vi "ArrangeNodes Main.vi"(1 "localVariablesOut":T1 {"ObjectHotspots"."HotSpot"."y" format="%.2f"; "ObjectHotspots"."HotSpot"."x" format="%.2f"; "NodesBounds"."height" format="%.2f"; "NodesBounds"."width" format="%.2f"; "NodesBounds"."y" format="%.2f"; "NodesBounds"."x" format="%.2f"; "offset"."y" format="%.2f"; "offset"."x" format="%.2f"; "gridSize" format="%.2f"; "dragStartBounds"."height" format="%.2f"; "dragStartBounds"."width" format="%.2f"; "dragStartBounds"."y" format="%.2f"; "dragStartBounds"."x" format="%.2f"; "dragStartPoint"."y" format="%.2f"; "dragStartPoint"."x" format="%.2f"; "rubberBandStart"."y" format="%.2f"; "rubberBandStart"."x" format="%.2f"; "lastMousePoint"."y" format="%.2f"; "lastMousePoint"."x" format="%.2f"; "zoom" format="%.2f"}) -> (15 "Cancel":bool)   [LabVIEW 2014]
uses:
  <resource>/Framework/Providers/Open_GDS/UML/UMLEditor/UMLEditor LocalVariablesType.ctl
  <resource>/Framework/Providers/Open_GDS/UML/Graphics_class/Graphics.lvclass
  <resource>/Framework/Providers/Open_GDS/UML/Grid_class/Grid.lvclass
  <resource>/Framework/Providers/Open_GDS/UML/AbstractEdge_class/AbstractEdge.lvclass
  <resource>/Framework/Providers/Open_GDS/UML/AbstractNode_class/AbstractNode.lvclass
  <resource>/Framework/Providers/Open_GDS/UML/UMLEditor/UMLEditor statesType.ctl
  <resource>/Framework/Providers/Open_GDS/UML/UMLEditor/UMLEditor tooltype.ctl
  <resource>/Framework/Providers/Open_GDS/UML/UMLEditor/UMLEditor toolsType.ctl
  <resource>/Framework/Providers/Open_GDS/UML/UMLEditor/UMLEditor_DiagramInfo.ctl
  <resource>/Framework/Providers/Open_GDS/UML/Graph_class/Graph.lvclass
  <resource>/Framework/Providers/Open_GDS/UML/General/Point/Point Point2D.ctl
  <resource>/Framework/Providers/Open_GDS/UML/General/Rectangle/Rectangle Rectangle2D.ctl
  <resource>/Framework/Providers/Open_GDS/UML/UMLEditor/UMLEditor ExportType.ctl
  <resource>/Framework/Providers/Open_GDS/UML/UMLEditor/UMLEditor FlattenCommandType.ctl
  <resource>/Framework/Providers/Open_GDS/UML/UMLEditor/UMLEditor ExecuteCommandType.ctl
  <resource>/Framework/Providers/Open_GDS/UML/ContextHelp/ContextHelp_EventType.ctl
  <resource>/Framework/Providers/Open_GDS/UML/UMLEditor/UMLEditor_HotSpotData.ctl
  <resource>/Framework/Providers/Open_GDS/UML/UMLEditor/UMLEditor_HotSpotType.ctl
  <resource>/Framework/Providers/Open_GDS/UML/UmlEditor_class/EventData.ctl
  <resource>/Framework/Providers/Open_GDS/UML/ArrangeNodes/private/ArrangeNodes LocalVar.ctl
  <resource>/Framework/Providers/Open_GDS/UML/ClassNode_class/ClassNode.lvclass
  <resource>/Framework/Providers/Open_GDS/UML/InterfaceNode_class/InterfaceNode.lvclass
  <resource>/Framework/Providers/Open_GDS/UML/StateNode_class/StateNode.lvclass
  <resource>/Framework/Providers/Open_GDS/UML/ContextHelp/ContextHelp_HelpTexts.ctl
  <resource>/Framework/Providers/Open_GDS/UML/MultiLineString_class/MultiLineString.lvclass
  <resource>/Framework/Providers/Open_GDS/UML/UmlEditor_class/UmlEditor.lvclass
panel:
  out "Picture":picture
  in  "Shake":bool
  in  "Help":bool
  in  "Zoom":enum16{"Normal", "Small", "Smaller", "Smallest"}(ring)
  in  "Auto Zoom":bool=TRUE
  in  "decrease":bool
  in  "OK":bool
  in  "Max Length":i32=350 min=10 max=1000
  in  "Min Length":i32=50 min=10 max=1000
  in  "increase":bool
  in  "shorten":bool
  in  "cancel":bool
  # "Left-Click and drag\na class.\n\nRight-click to lock/\nunlock class."
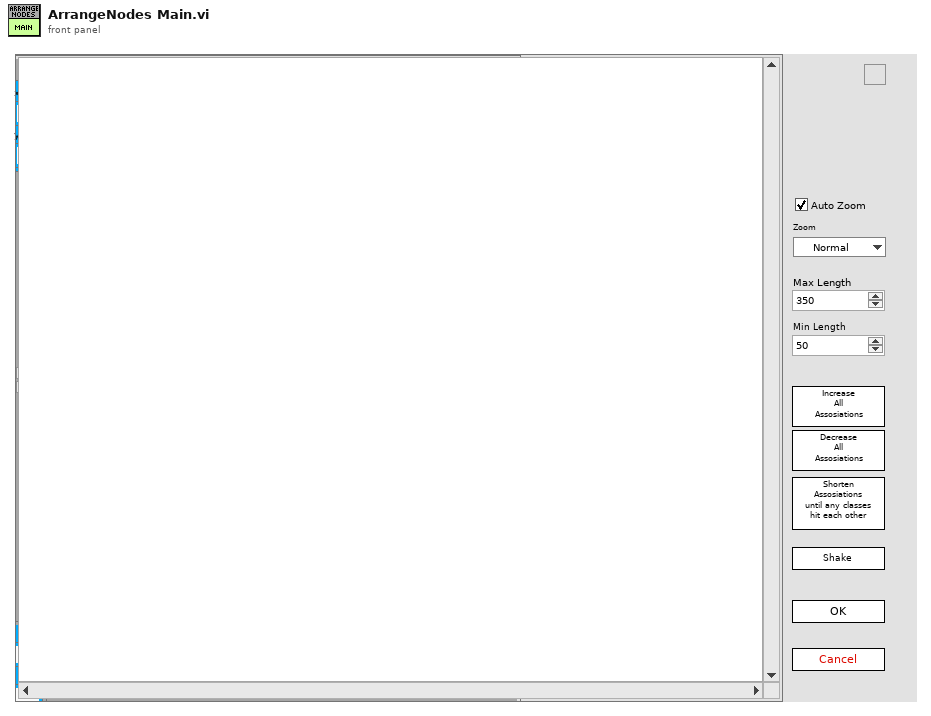
[diagram p1: front panel]
types:
  T1 = typedef "UMLEditor LocalVariablesType.ctl" = cluster{"state":T2, "graphics":refnum<class "Graphics.lvclass">, "grid":refnum<class "Grid.lvclass">, "toolType":T3, "tool":T4, "diagramIndex":i32, "diagrams":T5[], "zoom":dbl, "hideGrid":bool, "lastMousePoint":T6, "rubberBandStart":T6, "dragStartPoint":T6, "dragStartBounds":T7, "gridColor":u32, "gridSize":dbl, "CONNECT_THRESHOLD":i32, "selcted":T3, "selectedEdge":refnum<class "AbstractEdge.lvclass">, "butDwn":bool, "lastPress":u32, "modified":bool, "offset":T6, "menu":refnum<k9>, "file":path, "saveAs":bool, "newSelected":bool, "exportype":T8, "quit":bool, "revHistory":cluster{"rev":string, "text":string}[], "FlattenCommandSettings":T9, "PopUpMessageEvent":T11, "ResizePanelInProgress":bool, "NodesBounds":T7, "ToolHelp":bool, "ViRef":refnum<vi>, "FP_CtrlEnterEvents":refnum<event-registration>, "SelectedNodes":refnum<class "AbstractNode.lvclass">[], "mouse":refnum<k1>, "RevPlugInPath":path, "Action":string, "KeyPressTime":u32, "Cursors":refnum<k1>[], "ObjectHotspots":T12[], "HotSpotCursor":bool, "HotSpotFunction":T13, "Don'tDeleteChildren":bool, "ShiftDown":bool, "CtrlDown":bool, "HotSpotNode":refnum<class "AbstractNode.lvclass">, "Sync":bool, "SyncTime":u32, "ForceSyncNow":bool, "LastSync":timestamp, "XMI_Import":bool, "Event":refnum<event-registration>}
  T2 = typedef "UMLEditor statesType.ctl" = enum16{"Idle", "CheckLicense", "revHistory", "Init", "Init2", "EditSelected", "RemoveSelected", "PaintComponent", "ChangeZoom", "ChangeGridSize", "Open", "Close", "Save", "ExportPicture", "Export", "Repaint", "Error", "Exit", "QUIT", "CreateScript", "ExecuteScript", "ClassReversedEngineering", "PlugInReverseEngineering", "StateReversedEngineering", "AutoPlace", "ExecuteCommand", "OpenClass", "SyncAll", "StraightenAssociation", "Copy", "Paste", "AddNodeFromProjectTree", "AddNodeFromProjectTree+SyncAll", "PanAndRepaint", "Init3", "CopyPaste", "ApplyDesignPattern", "AnalyseViInStateDiagram", "AutoSync"}
  T3 = typedef "UMLEditor tooltype.ctl" = enum16{"None", "Node", "Edge"}
  T4 = typedef "UMLEditor toolsType.ctl" = enum16{"CD_Select", "CD_Class", "CD_Interface", "CD_Package", "CD_Note", "CD_Dependency", "CD_Inheritance", "CD_InterfaceImp", "CD_Association", "CD_Aggregation", "CD_Composite", "CD_NoteConn", "SQD_Select", "SQD_Object", "SQD_ActionBar", "SQD_Note", "SQD_Call", "SQD_NoteConn", "UD_Select", "UD_System", "UD_Actor", "UD_UseCase", "UD_Note", "UD_Assoiciation", "UD_Generalization", "UD_GeneralizationIncludes", "UD_GeneralizationExtends", "UD_Realization", "UD_Relationship", "UD_NoteEdge", "STD_Select", "STD_State", "STD_InitailState", "STD_FinalState", "STD_ChoiseState", "STD_StateTransation", "STD_Note", "STD_NoteEdge", "DM_Select", "DM_VI", "DM_Module", "DM_Request", "DM_RequestWait", "DM_Roundtrip", "DM_Broadcast", "DM_Note", "DM_NoteEdge"}
  T5 = typedef "UMLEditor_DiagramInfo.ctl" = cluster{"name":string, "diagramType":string, "unsaved":bool, "graph":refnum<class "Graph.lvclass">, "saveDir":path}
  T6 = typedef "Point Point2D.ctl" = cluster{"x":dbl, "y":dbl}
  T7 = typedef "Rectangle Rectangle2D.ctl" = cluster{"x":dbl, "y":dbl, "width":dbl, "height":dbl}
  T8 = typedef "UMLEditor ExportType.ctl" = enum16{"None", "Printer", "png", "jpg", "roseUML"}
  T9 = typedef "UMLEditor FlattenCommandType.ctl" = cluster{"Command":T10, "CommandData":variant}
  T10 = typedef "UMLEditor ExecuteCommandType.ctl" = enum16{"SyncUmlFromCode", "SyncCodeFromUML", "OpenClass", "OpenFile", "CreateClass", "CreateVI", "OpenClassAttribute", "LocateInProject"}
  T11 = typedef "ContextHelp_EventType.ctl" = refnum<user-event>
  T12 = typedef "UMLEditor_HotSpotData.ctl" = cluster{"Node":refnum<class "AbstractNode.lvclass">, "HotSpot":T6, "Function":T13}
  T13 = typedef "UMLEditor_HotSpotType.ctl" = enum16{"N", "NE", "E", "SE", "S", "SW", "W", "NW", "Expand", "Collaps"}
  T14 = typedef "ArrangeNodes LocalVar.ctl" = cluster{"nodes":cluster{"x":dbl, "y":dbl, "w":dbl, "h":dbl, "dx":dbl, "dy":dbl, "fixed":bool, "text":string, "maxCornerDist":dbl}[], "edges":cluster{"from":i32, "to":i32, "len":dbl}[], "nodeSelected":i32, "drag":bool, "NodeRef":u32[], "DragStart":cluster{"X":i32, "Y":i32}, "fixedBeforeDrag":bool, "Cancel":bool, "ClassNodes":refnum<class "AbstractNode.lvclass">[]}
  T15 = cluster{"bounds":T7, "className":string, "nodeRef":refnum<class "AbstractNode.lvclass">}[]
  T16 = cluster{"index of element":i32, "index of element":i32, bool}[]
  T17 = typedef "ContextHelp_HelpTexts.ctl" = enum16{"None(Hide)", "Default", "Help", "Welcome", "GettingStarted", "ClassDiagram_Help", "SequenceDiagram_Help", "UseCaseDiagram_Help", "BSelect", "BClass", "BInterface", "BPackage", "BNote", "BDependency", "BInheritance", "BInterfaceImplementation", "BAssociation", "BAggregation", "BCompAggregation", "BNoteConnector", "BObject", "BActionBar", "BCall", "BSystem", "BActor", "BUseCase", "BGeneralization", "BIncludes", "BExtends", "BUseCaseDiagramAssociation", "ClassRelationshipEdge editDialog_Bent Style", "ClassRelationshipEdge editDialog_RelationType", "ClassRelationshipEdge editDialog_Reverse association", "ClassRelationshipEdge editDialog_Start label", "ClassRelationshipEdge editDialog_Middle label", "ClassRelationshipEdge editDialog_End label", "UMLEditor reversedEngineering_Pathes", "ReversedEngineering StateReverseDialog_Help", "ReversedEngineering StateQueuedSettings_Help", "UMLEditor reversedEngineering_AddTopVIs", "UMLEditor reversedEngineering_AddClasses", "UMLEditor reversedEngineering_AddDirs", "UMLEditor reversedEngineering_Recursively", "UMLEditor reversedEngineering_Remove", "UMLEditor reversedEngineering_ClearList", "UMLEditor reversedEngineering_HideSubAss", "UMLEditor reversedEngineering_CreateTypes", "UMLEditor reversedEngineering_OnlyInheritance", "UMLEditor reversedEngineering_CreateApplication", "UMLEditor reversedEngineering_OK", "UMLEditor reversedEngineering_Cancel", "UMLEditor reversedEngineering_Help", "UMLEditor createWizardScriptFile_ScriptfilePath", "UMLEditor createWizardScriptFile_ClassPath", "UMLEditor createWizardScriptFile_Use", "UMLEditor createWizardScriptFile_PrivateDirName", "UMLEditor createWizardScriptFile_DirAppend", "UMLEditor createWizardScriptFile_Separator Character", "UMLEditor createWizardScriptFile_OK", "UMLEditor createWizardScriptFile_Cancel", "UMLEditor createWizardScriptFile_Help", "ClassNode editDialog_Class Name", "InterfaceNode editDialog_Class Name", "ClassNode editDialog_Attribute", "ClassNode editDialog_Methods", "InterfaceNode editDialog_Methods", "ClassNode editDialog_connection", "InterfaceNode editDialog_connection", "ClassNode editDialog_StereoType", "ClassNode editDialog_ShowAttrib", "ClassNode editDialog_ShowMethods", "ClassNode editDialog_ClassPath", "ClassNode editDialog_AddAttribute", "ClassNode editDialog_AddMethod", "InterfaceNode editDialog_AddMethod", "ClassNode AttributeGuide_AttributeName", "ClassNode AttributeGuide_Array?", "ClassNode AttributeGuide_Data Type", "ClassNode AttributeGuide_RefName", "ClassNode AttributeGuide_Preview", "ClassNode AttributeGuide_OK", "ClassNode AttributeGuide_Cancel", "ClassNode MethodGuide_Visibility", "ClassNode MethodGuide_Method Name", "ClassNode MethodGuide_Preview", "ClassNode MethodGuide_OK", "ClassNode MethodGuide_Cancel", "CallNode EditCallProperties_AllButtons", "ObjectNode EditObjectlProperties_AllButtons", "ActorNode EditActorProperties_AllButtons", "UseCaseRelationshipNode EditUseCaselProperties_AllButtons", "UseCaseNode EditUseCaselProperties_AllButtons", "SystemNode EditSystemProperties_AllButtons", "ReversedEngineering UpdateAttributes_AllButtons", "StateNode editDialog_AllButtons", "StateTransition editDialog_AllButtons", "ArrangeNodes Main_Picture", "ArrangeNodes Main_Zoom", "ArrangeNodes Main_Auto Zoom", "ArrangeNodes Main_shorten", "ArrangeNodes Main_Min Length", "ArrangeNodes Main_Max Length", "ArrangeNodes Main_increase", "ArrangeNodes Main_decrease", "ArrangeNodes Main_Shake", "ArrangeNodes Main", "BState", "BInitialState", "BFinalState", "BStateTransition", "StateDiagram_Help", "StateDiagram_PropertiesAllButtons", "ReversedEngineering StateReverseDialog_ClearStates", "ReversedEngineering StateReverseDialog_UseQueuedStateMachines", "ReversedEngineering StateReverseDialog_QueuedSettings", "ReversedEngineering StateReverseDialog_SearchForVIs", "ReversedEngineering StateReverseDialog_SearchCriteria", "OptionsDialog_ClassBasePath", "OptionsDialog_VIPath", "OptionsDialog_ApplicationPath", "OptionsDialog_WizDir", "OptionsDialog_IniFilePath", "OptionsDialog_DefineColors", "OptionsDialog_Help", "OptionsDialog_CreateTypes", "ClassRelationshipEdge editDialog_SplitWire"}
  T18 = cluster{"bounds":T7, "text":string, "reference out":refnum<class "AbstractNode.lvclass">}
  T19 = cluster{"bounds":T7, "text":string, "reference out":refnum<class "AbstractNode.lvclass">}[]
  T20 = cluster{"x":dbl, "y":dbl, "w":dbl, "h":dbl, "dx":dbl, "dy":dbl, "fixed":bool, "text":string, "maxCornerDist":dbl}[]
  T21 = cluster{"x":dbl, "y":dbl, "w":dbl, "h":dbl, "dx":dbl, "dy":dbl, "fixed":bool, "text":string, "maxCornerDist":dbl}
  T22 = cluster{"index of element":i32, "index of element":i32, "isInheritance":bool}
  T23 = cluster{"index of element":i32, "index of element":i32, "isInheritance":bool}[]
  T24 = typedef "LVMouseTypeDef.ctl" = cluster{"Mouse Position":cluster{"X":i32, "Y":i32}, "Mouse Modifiers":cluster{"Button Down":bool, "Shift Mod":bool, "Menu Mod":bool, "Option Mod":bool}}
  T25 = typedef "ContextHelp_ShowType.ctl" = cluster{"Header":string, "Picture":picture, "Text":string}
  T26 = typedef "LVBoundsTypeDef.ctl" = cluster{"Width":u32, "Height":u32}
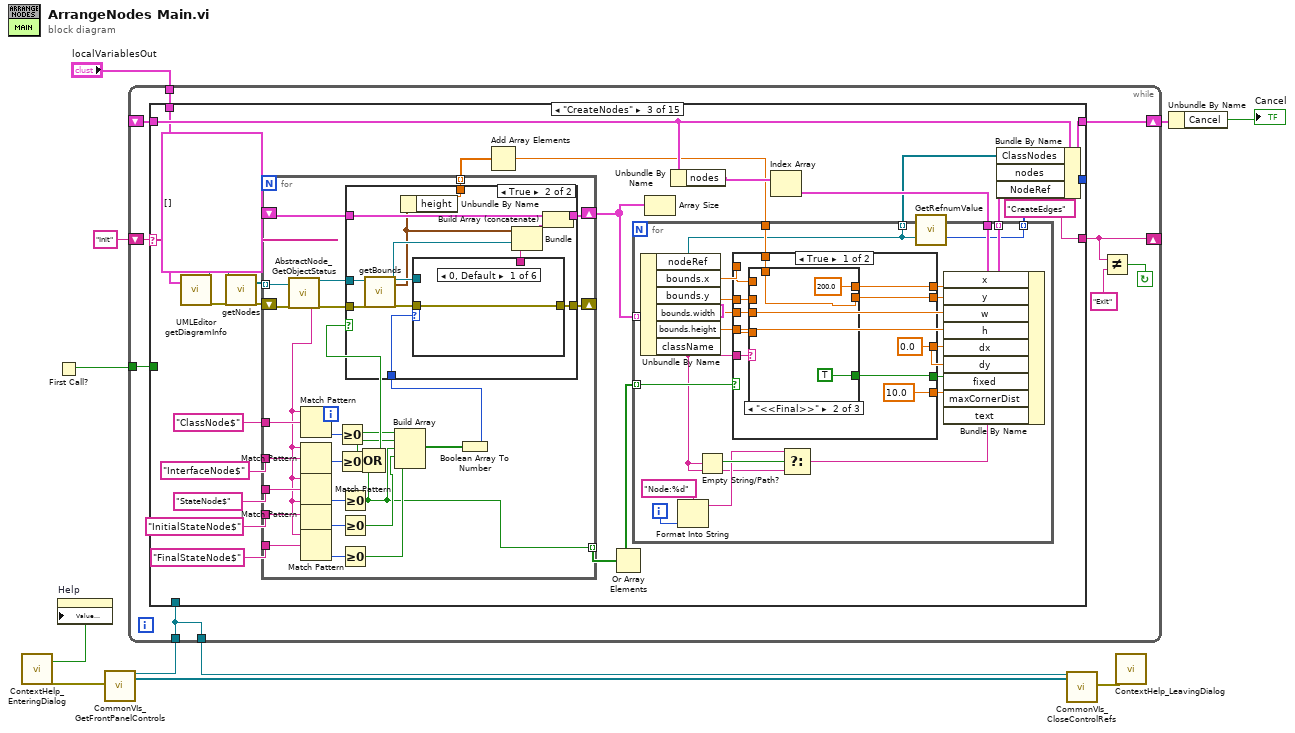
[diagram p0: block diagram]
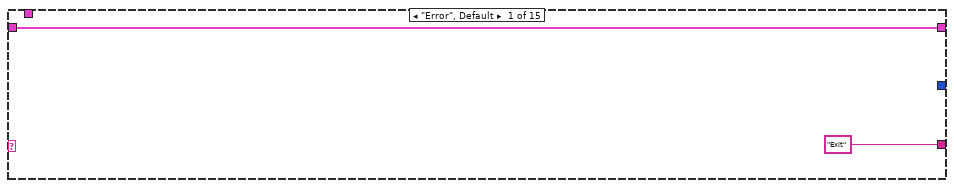
[diagram p2: hidden frame]
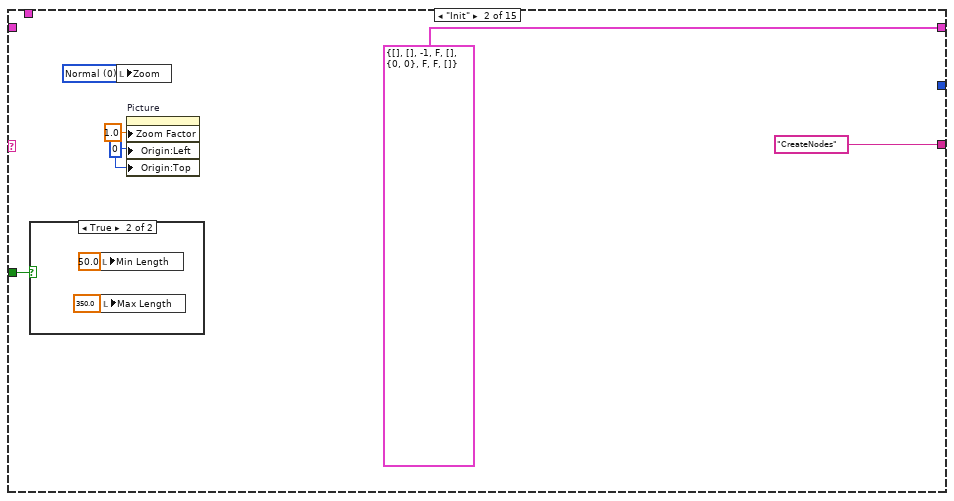
[diagram p3: hidden frame]
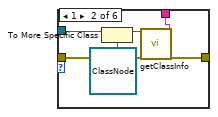
[diagram p6: hidden frame]
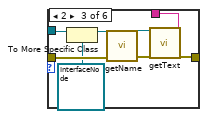
[diagram p7: hidden frame]
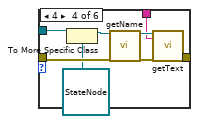
[diagram p8: hidden frame]
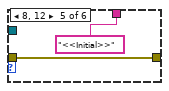
[diagram p9: hidden frame]
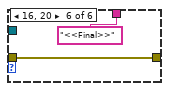
[diagram p10: hidden frame]
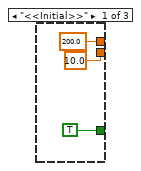
[diagram p11: hidden frame]
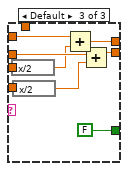
[diagram p12: hidden frame]
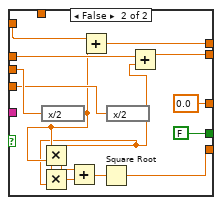
[diagram p13: hidden frame]
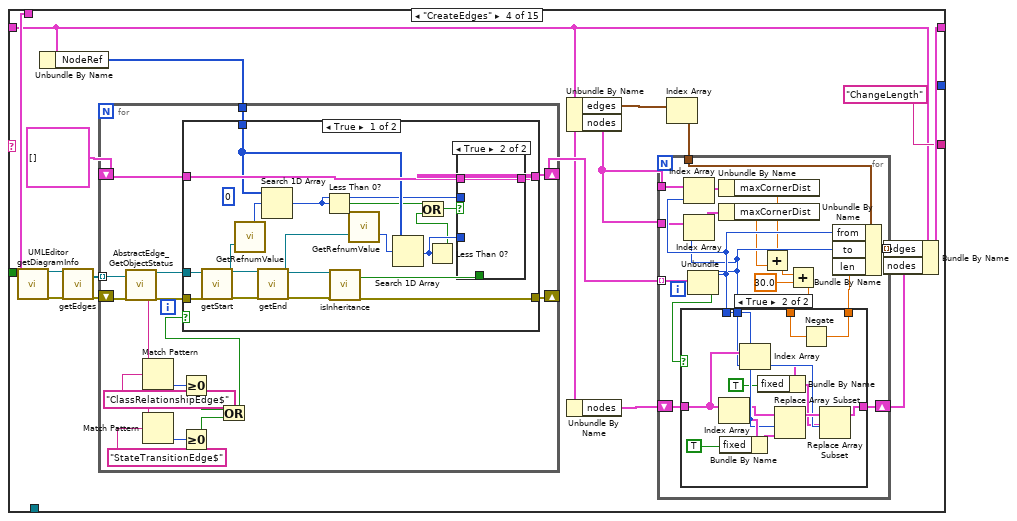
[diagram p14: hidden frame]
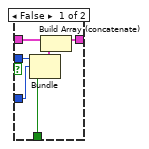
[diagram p15: hidden frame]
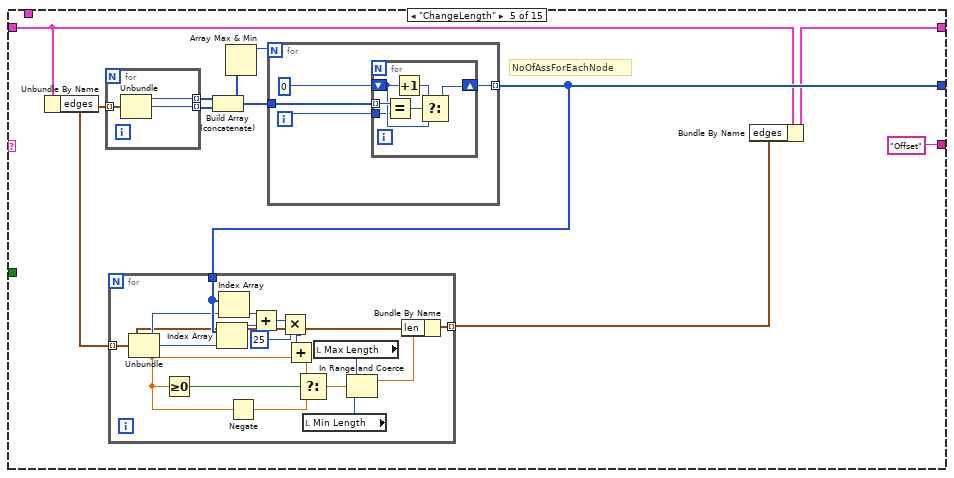
[diagram p18: hidden frame]
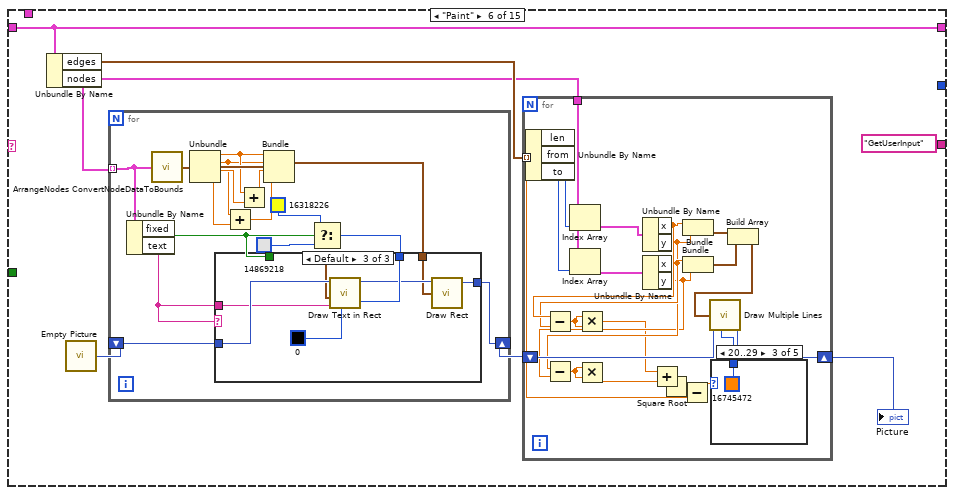
[diagram p19: hidden frame]
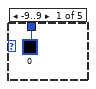
[diagram p20: hidden frame]
diagram:
  n1 = call <resource>:"ContextHelp_EnteringDialog.vi"() -> ("HelpStatus"=w3:bool, "error out"=w6:errorcluster)  [unwired: 3 in, 15 out]
  n2 = First Call?() -> (First Call?: T/F=w9:bool)
  n3 = property on="Help" class="Bool (strict)"("Value (Signaling)"=w3) -> ()  [unwired: 2 in, 2 out]
  n4 = call <resource>:"CommonVIs_GetFrontPanelControls.vi"("error in (no error)"=w6) -> ("Event Registration Refnum"=w5:refnum<event-registration>, "ControlRefs"=w8:refnum<vi>[])  [unwired: 1 in, 16 out]
  n5 = while {
    shift-left: _ -> [w15]
    shift-right: [w16] -> w2
    shift-left: "Init" -> [w20]
    shift-right: [w18] -> _
    tunnel: "localVariablesOut" -> [w14]
    tunnel: w9 -> [w13]
    tunnel: w5 -> [w12]
    tunnel: [w12] -> w4
    stop <- w19 continue-if-true
    n6 = case shown="\"CreateNodes\"" w20 {
      tunnel: ["Exit" "CreateNodes" "CreateEdges" "ChangeLength" "Offset" "GetUserInput" w403 "Paint" "Paint" "Paint" "Paint" "Paint" "Offset" "Paint" "Exit"] -> w18
      tunnel: [w21 T14 {"nodes"=[], "edges"=[], "nodeSelected"=-1, "drag"=FALSE, "NodeRef"=[], "DragStart"={"X"=0, "Y"=0}, "fixedBeforeDrag"=FALSE, "Cancel"=FALSE, "ClassNodes"=[]} ("Cluster") w50 w198 w280 w321 w405 w586 w633 w722 w778 w791 w804 w831 w905] -> w16
      tunnel: w15 -> [w21 _ w51 w187 w281 w321 w404 w587 w636 w723 w779 w792 w805 w832 w905]
      tunnel: w14 -> [_ _ w43 w191 _ _ _ _ _ _ _ _ _ _ _]
      tunnel: w13 -> [_ w26 _ _ _ _ _ _ _ _ _ _ _ _ _]
      tunnel: [_ _ _ _ w282 _ _ _ _ _ _ _ _ _ _] -> _
      tunnel: w12 -> [_ _ _ _ _ _ w398 _ _ _ _ _ _ _ _]
      frame "Error", Default {
      }
      frame "Init" {
        w23 = i16 0 ("Origin:Left")
        w24 = u16 0 items=["Normal", "Small", "Smaller", "Smallest"] ("Zoom")
        n7 = case shown="True" w26 {
          frame False {
          }
          frame True {
            n8 = local write "Min Length"(50.0 ("Min Length")) -> ()
            n9 = local write "Max Length"(350.0 ("Max Length")) -> ()
          }
        }
        n10 = local write "Zoom"(w24) -> ()
        n11 = property on="Picture" class="Pict"("Zoom Factor"=sgl 1.0, "Origin:Left"=w23, "Origin:Top"=w23) -> ()  [unwired: 2 in, 2 out]
      }
      frame "CreateNodes" {
        n12 = call <resource>:"UMLEditor getDiagramInfo.vi"("localVariables"=w43) -> ("graph"=w44:refnum<class "Graph.lvclass">, "error out"=w45:errorcluster)  [unwired: 1 in, 16 out]
        n13 = call-dynamic "getNodes.vi"("reference"=w44, "error in (no error)"=w45) -> ("nodes"=w46:refnum<class "AbstractNode.lvclass">[], "error out"=w47:errorcluster)  [unwired: 15 in, 1 out]
        n14 = for {
          tunnel: w46 -> [w79] mode=indexing
          shift-right: [w74] -> _
          shift-left: w47 -> [w80]
          shift-right: [w75] -> w34
          shift-left: T15 [] -> [w76]
          tunnel: "ClassNode$" ("y") -> [w71]
          tunnel: "InterfaceNode$" ("y") -> [w70]
          tunnel: "StateNode$" ("y") -> [w69]
          tunnel: "InitialStateNode$" ("y") -> [w63]
          tunnel: "FinalStateNode$" ("y") -> [w62]
          tunnel: [w55] -> w35 mode=indexing
          tunnel: [w54] -> w33 mode=indexing
          n15 = call <resource>:"AbstractNode_GetObjectStatus.vi"("reference in"=w79, "error in (no error)"=w80) -> ("Class name"=w56:string, "reference out"=w77:refnum<class "AbstractNode.lvclass">, "error out"=w78:errorcluster)  [unwired: 15 out]
          n16 = Match Pattern(string=w56, regular expression=w71) -> (offset past match=w72:i32)  [unwired: 4 out]
          n17 = Match Pattern(string=w56, regular expression=w70) -> (offset past match=w73:i32)  [unwired: 4 out]
          n18 = Match Pattern(string=w56, regular expression=w69) -> (offset past match=w68:i32)  [unwired: 4 out]
          n19 = Match Pattern(string=w56, regular expression=w63) -> (offset past match=w64:i32)  [unwired: 4 out]
          n20 = Match Pattern(string=w56, regular expression=w62) -> (offset past match=w61:i32)  [unwired: 4 out]
          n21 = Greater Or Equal To 0?(x=w72) -> (x >= 0?=w66:bool)
          n22 = Greater Or Equal To 0?(x=w73) -> (x >= 0?=w65:bool)
          n23 = Greater Or Equal To 0?(x=w68) -> (x >= 0?=w55:bool)
          n24 = Greater Or Equal To 0?(x=w64) -> (x >= 0?=w60:bool)
          n25 = Greater Or Equal To 0?(x=w61) -> (x >= 0?=w59:bool)
          n26 = Compound Arithmetic op=OR(w66, w65, w55) -> (w67:bool)
          n27 = Build Array(w66, w65, w55, w60, w59) -> (w58:bool[])
          n28 = Boolean Array To Number(Boolean array=w58) -> (number=w57:u32)
          n29 = case shown="True" w67 {
            tunnel: w78 -> [w81 w94]
            tunnel: w77 -> [_ w93]
            tunnel: w76 -> [w82 w92]
            tunnel: [w82 w91] -> w75
            tunnel: [w81 w87] -> w74
            tunnel: w57 -> [_ w86]
            tunnel: [_ w83] -> w54
            frame False {
            }
            frame True {
              n30 = call-dynamic "getBounds.vi"("reference"=w93, "error in (no error)"=w94) -> ("reference out"=w85:refnum<class "AbstractNode.lvclass">, "bounds"=w84:T7, "error out"=w89:errorcluster)  [unwired: 15 in]
              n31 = Unbundle By Name(w84) -> ("height"=w83:dbl)
              n32 = case shown="0, Default" w86 {
                tunnel: w89 -> [w95 w99 w109 w117 w118 w120]
                tunnel: w85 -> [_ w98 w104 w112 _ _]
                tunnel: [_ w101 w105 w113 "<<Initial>>" "<<Final>>"] -> w88
                tunnel: [w95 w100 w106 w114 w118 w120] -> w87
                frame 0, Default {
                }
                frame 1 {
                  n33 = To More Specific Class(target class=refnum<class "ClassNode.lvclass"> refnum ("reference"), reference=w98) -> (specific class reference=w97:refnum<class "ClassNode.lvclass">)  [unwired: 1 in, 1 out]
                  n34 = call-dynamic "getClassInfo.vi"("reference"=w97, "error in (no error)"=w99) -> ("className"=w101:string, "error out"=w100:errorcluster)  [unwired: 8 in, 8 out]
                }
                frame 2 {
                  n35 = To More Specific Class(target class=refnum<class "InterfaceNode.lvclass"> refnum ("reference"), reference=w104) -> (specific class reference=w103:refnum<class "InterfaceNode.lvclass">)  [unwired: 1 in, 1 out]
                  n36 = call-dynamic "getName.vi"("reference"=w103, "error in (no error)"=w109) -> ("name"=w108:refnum<class "MultiLineString.lvclass">, "error out"=w107:errorcluster)  [unwired: 15 in, 1 out]
                  n37 = call-dynamic "getText.vi"("reference"=w108, "error in (no error)"=w107) -> ("text"=w105:string, "error out"=w106:errorcluster)  [unwired: 15 in, 1 out]
                }
                frame 4 {
                  n38 = To More Specific Class(target class=refnum<class "StateNode.lvclass"> refnum ("reference"), reference=w112) -> (specific class reference=w111:refnum<class "StateNode.lvclass">)  [unwired: 1 in, 1 out]
                  n39 = call-dynamic "getName.vi"("reference"=w111, "error in (no error)"=w117) -> ("name"=w116:refnum<class "MultiLineString.lvclass">, "error out"=w115:errorcluster)  [unwired: 15 in, 1 out]
                  n40 = call-dynamic "getText.vi"("reference"=w116, "error in (no error)"=w115) -> ("text"=w113:string, "error out"=w114:errorcluster)  [unwired: 15 in, 1 out]
                }
                frame 8, 12 {
                }
                frame 16, 20 {
                }
              }
              n41 = Bundle("bounds"=w84, "text"=w88, "reference out"=w85) -> (w90:T18)  [unwired: 1 out]
              n42 = Build Array (concatenate)(w92, w90) -> (w91:T19)
            }
          }
        }
        n43 = Add Array Elements(numeric array=w33) -> (sum=w32:dbl)
        n44 = Or Array Elements(Boolean array=w35) -> ()  [unwired: 1 out]
        n45 = Array Size(array=w34) -> ()  [unwired: 1 out]
        n46 = Unbundle By Name(w51) -> ("nodes"=w53:T20)
        n47 = Index Array(array=w53) -> (element=w52:T21)  [unwired: 1 in]
        n48 = for {
          tunnel: w52 -> [w143]
          tunnel: [w138] -> w49 mode=indexing
          tunnel: w34 -> [w137] mode=indexing
          tunnel: [w123] -> w41 mode=indexing
          tunnel: w35 -> [w126] mode=indexing
          tunnel: w32 -> [w124]
          tunnel: [w122] -> w31 mode=indexing
          i -> [w140]
          n49 = Unbundle By Name(w137) -> ("nodeRef"=w122:refnum<class "AbstractNode.lvclass">, "bounds.x"=w133:dbl, "bounds.y"=w131:dbl, "bounds.width"=w129:dbl, "bounds.height"=w128:dbl, "className"=w125:string)
          n50 = Format Into String(format string="Node:%d" ("Format String"), w140) -> (resulting string=w135:string)  [unwired: 2 in, 1 out]
          n51 = Empty String/Path?(string/path=w125) -> (empty?=w136:bool)
          n52 = case shown="True" w126 {
            tunnel: [w144 FALSE ("fixed")] -> w142
            tunnel: [0.0 ("dx") 0.0 ("dx")] -> w141
            tunnel: w133 -> [w153 w181]
            tunnel: [w152 w180] -> w132
            tunnel: w131 -> [w151 w179]
            tunnel: [w150 w178] -> w130
            tunnel: w129 -> [w149 w177]
            tunnel: w128 -> [w148 w176]
            tunnel: [10.0 ("dx") w172] -> w127
            tunnel: w125 -> [w146 _]
            tunnel: w124 -> [w145 _]
            frame True {
              n53 = case shown="\"<<Final>>\"" w146 {
                tunnel: w153 -> [_ _ w169]
                tunnel: [200.0 200.0 w168] -> w152
                tunnel: w151 -> [_ _ w167]
                tunnel: [10.0 w159 w166] -> w150
                tunnel: w149 -> [_ _ w165]
                tunnel: w148 -> [_ _ w164]
                tunnel: w145 -> [_ w159 _]
                tunnel: [TRUE ("fixed") TRUE ("fixed") FALSE ("fixed")] -> w144
                frame "<<Initial>>" {
                }
                frame "<<Final>>" {
                }
                frame Default {
                  n54 = expression code="x/2"(w165) -> (w163:dbl)
                  n55 = expression code="x/2"(w164) -> (w162:dbl)
                  n56 = Add(x=w169, y=w163) -> (x+y=w168:dbl)
                  n57 = Add(x=w167, y=w162) -> (x+y=w166:dbl)
                }
              }
            }
            frame False {
              n58 = expression code="x/2"(w177) -> (w171:dbl)
              n59 = Multiply(x=w171, y=w171) -> (x*y=w175:dbl)
              n60 = Add(x=w181, y=w171) -> (x+y=w180:dbl)
              n61 = expression code="x/2"(w176) -> (w170:dbl)
              n62 = Multiply(x=w170, y=w170) -> (x*y=w174:dbl)
              n63 = Add(x=w175, y=w174) -> (x+y=w173:dbl)
              n64 = Square Root(x=w173) -> (sqrt(x)=w172:dbl)
              n65 = Add(x=w179, y=w170) -> (x+y=w178:dbl)
            }
          }
          n66 = Select(t=w135, s=w136, f=w125) -> (s? t:f=w134:string)
          n67 = call <resource>:"GetRefnumValue.vi"("reference"=w122) -> ("RefNum"=w123:i32)  [unwired: 17 in, 1 out]
          n68 = Bundle By Name(cluster=w143, "x"=w132, "y"=w130, "w"=w129, "h"=w128, "dx"=w141, "dy"=w141, "fixed"=w142, "maxCornerDist"=w127, "text"=w134) -> (w138:T21)
        }
        n69 = Bundle By Name(cluster=w51, "ClassNodes"=w31, "nodes"=w49, "NodeRef"=w41) -> (w50:T14)
      }
      frame "CreateEdges" {
        n70 = call <resource>:"UMLEditor getDiagramInfo.vi"("localVariables"=w191) -> ("graph"=w192:refnum<class "Graph.lvclass">, "error out"=w193:errorcluster)  [unwired: 1 in, 16 out]
        n71 = Unbundle By Name(w187) -> ("NodeRef"=w190:u32[])
        n72 = call-dynamic "getEdges.vi"("reference"=w192, "error in (no error)"=w193) -> ("edges"=w194:refnum<class "AbstractEdge.lvclass">[], "error out"=w195:errorcluster)  [unwired: 15 in, 1 out]
        n73 = for {
          tunnel: w194 -> [w215] mode=indexing
          shift-right: [w210] -> _
          shift-left: w195 -> [w216]
          shift-right: [w211] -> w188
          shift-left: T16 [] -> [w212]
          tunnel: w190 -> [w209]
          n74 = call <resource>:"AbstractEdge_GetObjectStatus.vi"("reference in"=w215, "error in (no error)"=w216) -> ("Class name"=w207:string, "reference out"=w213:refnum<class "AbstractEdge.lvclass">, "error out"=w214:errorcluster)  [unwired: 9 in, 6 out]
          n75 = Match Pattern(string=w207, regular expression="ClassRelationshipEdge$" ("y")) -> (offset past match=w205:i32)  [unwired: 4 out]
          n76 = Match Pattern(string=w207, regular expression="StateTransitionEdge$" ("y")) -> (offset past match=w204:i32)  [unwired: 4 out]
          n77 = Greater Or Equal To 0?(x=w205) -> (x >= 0?=w202:bool)
          n78 = Greater Or Equal To 0?(x=w204) -> (x >= 0?=w203:bool)
          n79 = Or(x=w202, y=w203) -> (x .or. y?=w201:bool)
          n80 = case shown="True" w201 {
            tunnel: w214 -> [w236 w244]
            tunnel: w213 -> [w235 _]
            tunnel: w212 -> [w234 w245]
            tunnel: [w233 w245] -> w211
            tunnel: [w224 w244] -> w210
            tunnel: w209 -> [w230 _]
            frame True {
              (unwired) u32 0
              n81 = call-dynamic "getStart.vi"("reference"=w235, "error in (no error)"=w236) -> ("reference out"=w231:refnum<class "AbstractEdge.lvclass">, "startNode"=w220:refnum<class "AbstractNode.lvclass">, "error out"=w232:errorcluster)  [unwired: 14 in, 1 out]
              n82 = call <resource>:"GetRefnumValue.vi"("reference"=w220) -> ("RefNum"=w219:i32)  [unwired: 17 in, 1 out]
              n83 = call-dynamic "getEnd.vi"("reference"=w231, "error in (no error)"=w232) -> ("reference out"=w223:refnum<class "AbstractEdge.lvclass">, "endNode"=w218:refnum<class "AbstractNode.lvclass">, "error out"=w225:errorcluster)  [unwired: 14 in, 1 out]
              n84 = Search 1D Array(1D array=w230, element=w219) -> (index of element=w227:i32)  [unwired: 1 out]
              n85 = Less Than 0?(x=w227) -> (x < 0?=w229:bool)
              n86 = call-dynamic "isInheritance.vi"("reference"=w223, "error in (no error)"=w225) -> ("isInheritance"=w221:bool, "error out"=w224:errorcluster)  [unwired: 14 in, 2 out]
              n87 = call <resource>:"GetRefnumValue.vi"("reference"=w218) -> ("RefNum"=w217:i32)  [unwired: 17 in, 1 out]
              n88 = Search 1D Array(1D array=w230, element=w217) -> (index of element=w226:i32)  [unwired: 1 out]
              n89 = Less Than 0?(x=w226) -> (x < 0?=w222:bool)
              n90 = Or(x=w229, y=w222) -> (x .or. y?=w228:bool)
              n91 = case shown="True" w228 {
                tunnel: w234 -> [w242 w243]
                tunnel: [w241 w243] -> w233
                tunnel: w227 -> [w240 _]
                tunnel: w226 -> [w239 _]
                tunnel: w221 -> [w237 _]
                frame False {
                  n92 = Bundle("index of element"=w240, "index of element"=w239, "isInheritance"=w237) -> (w238:T22)  [unwired: 1 out]
                  n93 = Build Array (concatenate)(w242, w238) -> (w241:T23)
                }
                frame True {
                }
              }
            }
            frame False {
            }
          }
        }
        n94 = Unbundle By Name(w187) -> ("edges"=w200:cluster{"from":i32, "to":i32, "len":dbl}[], "nodes"=w184:T20)
        n95 = Unbundle By Name(w187) -> ("nodes"=w186:T20)
        n96 = Index Array(array=w200) -> (element=w199:cluster{"from":i32, "to":i32, "len":dbl})  [unwired: 1 in]
        n97 = for {
          tunnel: w199 -> [w263]
          tunnel: [w262] -> w197 mode=indexing
          tunnel: w188 -> [w261] mode=indexing
          shift-right: [w259] -> w185
          shift-left: w186 -> [w260]
          tunnel: w184 -> [w255]
          tunnel: w184 -> [w254]
          n98 = Unbundle(w261) -> ("index of element"=w257:i32, "index of element"=w256:i32, w258:bool)
          n99 = Index Array(array=w255, index=w257) -> (element=w253:T21)
          n100 = Index Array(array=w254, index=w256) -> (element=w252:T21)
          n101 = Unbundle By Name(w253) -> ("maxCornerDist"=w250:dbl)
          n102 = Unbundle By Name(w252) -> ("maxCornerDist"=w251:dbl)
          n103 = Add(x=w250, y=w251) -> (x+y=w248:dbl)
          n104 = Add(x=w248, y=30.0) -> (x+y=w246:dbl)
          n105 = case shown="True" w258 {
            tunnel: w260 -> [w265 w276]
            tunnel: w257 -> [_ w277]
            tunnel: w256 -> [_ w272]
            tunnel: [w265 w268] -> w259
            tunnel: [w264 w266] -> w249
            tunnel: w246 -> [w264 w267]
            frame False {
            }
            frame True {
              n106 = Index Array(array=w276, index=w277) -> (element=w278:T21)
              n107 = Bundle By Name(cluster=w278, "fixed"=TRUE) -> (w275:T21)
              n108 = Index Array(array=w276, index=w272) -> (element=w270:T21)
              n109 = Bundle By Name(cluster=w270, "fixed"=TRUE) -> (w269:T21)
              n110 = Replace Array Subset(array=w276, new element=w275, index=w277) -> (w273:T20)
              n111 = Negate(x=w267) -> (-x=w266:dbl)
              n112 = Replace Array Subset(array=w273, new element=w269, index=w272) -> (w268:T20)
            }
          }
          n113 = Bundle By Name(cluster=w263, "from"=w257, "to"=w256, "len"=w249) -> (w262:cluster{"from":i32, "to":i32, "len":dbl})
        }
        n114 = Bundle By Name(cluster=w187, "edges"=w197, "nodes"=w185) -> (w198:T14)
      }
      frame "ChangeLength" {
        # "NoOfAssForEachNode"
        n115 = Unbundle By Name(w281) -> ("edges"=w283:cluster{"from":i32, "to":i32, "len":dbl}[])
        n116 = for {
          tunnel: w283 -> [w319] mode=indexing
          tunnel: [w318] -> w288 mode=indexing
          tunnel: [w317] -> w287 mode=indexing
          n117 = Unbundle(w319) -> ("from"=w318:i32, "to"=w317:i32)  [unwired: 1 out]
        }
        n118 = Build Array (concatenate)(w288, w287) -> (w286:i32[])
        n119 = Array Max & Min(array=w286) -> (max value=w285:i32)  [unwired: 3 out]
        n120 = for {
          N: w285 -> [_]
          tunnel: w286 -> [w310]
          tunnel: [w307] -> w282 mode=indexing
          i -> [w309]
          n121 = for {
            tunnel: w310 -> [w316] mode=indexing
            shift-right: [w313] -> w307
            shift-left: 0 -> [w312]
            tunnel: w309 -> [w311]
            n122 = Equal?(x=w316, y=w311) -> (x = y?=w315:bool)
            n123 = Increment(x=w312) -> (x+1=w314:i32)
            n124 = Select(t=w314, s=w315, f=w312) -> (s? t:f=w313:i32)
          }
        }
        n125 = for {
          tunnel: w283 -> [w300] mode=indexing
          tunnel: w282 -> [w306]
          tunnel: [w299] -> w279 mode=indexing
          n126 = Unbundle(w300) -> ("from"=w305:i32, "to"=w304:i32, "len"=w289:dbl)
          n127 = Greater Or Equal To 0?(x=w289) -> (x >= 0?=w301:bool)
          n128 = Index Array(array=w306, index=w304) -> (element=w302:i32)
          n129 = Index Array(array=w306, index=w305) -> (element=w303:i32)
          n130 = Negate(x=w289) -> (-x=w291:dbl)
          n131 = Add(x=w303, y=w302) -> (x+y=w298:i32)
          n132 = Multiply(x=w298, y=25) -> (x*y=w296:i32)
          n133 = Add(x=w296, y=w289) -> (x+y=w290:dbl)
          n134 = Select(t=w290, s=w301, f=w291) -> (s? t:f=w295:dbl)
          n135 = local read "Min Length"() -> (w294:i32)
          n136 = local read "Max Length"() -> (w293:i32)
          n137 = In Range and Coerce(upper limit=w293, x=w295, lower limit=w294) -> (coerced(x)=w292:dbl)  [unwired: 1 out]
          n138 = Bundle By Name(cluster=w300, "len"=w292) -> (w299:cluster{"from":i32, "to":i32, "len":dbl})
        }
        n139 = Bundle By Name(cluster=w281, "edges"=w279) -> (w280:T14)
      }
      frame "Paint" {
        n140 = Unbundle By Name(w321) -> ("edges"=w324:cluster{"from":i32, "to":i32, "len":dbl}[], "nodes"=w323:T20)
        n141 = call "Empty Picture"() -> ("empty picture"=w326:picture)
        n142 = for {
          tunnel: w323 -> [w367] mode=indexing
          shift-right: [w366] -> w325
          shift-left: w326 -> [w368]
          n143 = Unbundle By Name(w367) -> ("fixed"=w356:bool, "text"=w357:string)
          n144 = call <resource>:"ArrangeNodes ConvertNodeDataToBounds.vi"("NodeData"=w367) -> ("NodeBounds"=w365:cluster{"x":dbl, "y":dbl, "w":dbl, "h":dbl})
          n145 = Unbundle(w365) -> ("x"=w362:dbl, "y"=w359:dbl, "w"=w361:dbl, "h"=w358:dbl)
          n146 = Add(x=w359, y=w358) -> (x+y=w360:dbl)
          n147 = Add(x=w362, y=w361) -> (x+y=w363:dbl)
          n148 = Bundle(cluster=w365, "x"=w362, "y"=w359, "w"=w363, "h"=w360) -> (w364:cluster{"x":dbl, "y":dbl, "w":dbl, "h":dbl})
          n149 = Select(t=u32 16318226, s=w356, f=u32 14869218) -> (s? t:f=w369:u32)
          n150 = case shown="Default" w357 {
            tunnel: w369 -> [_ _ w397]
            tunnel: w368 -> [w375 w388 w396]
            tunnel: w357 -> [_ _ w394]
            tunnel: [w382 w389 w392] -> w366
            tunnel: w364 -> [w373 w390 w391]
            tunnel: w356 -> [w380 w386 _]
            frame "<<Final>>" {
              n151 = Select(t=u32 16318226, s=w380, f=u32 0) -> (s? t:f=w372:u32)
              n152 = call <vilib>:"Draw Oval.vi"("picture"=w375, "rect"=w373, "color(black)"=w372) -> ("new picture"=w374:picture)  [unwired: 2 in, 4 out]
              n153 = Add(x=w373, y=cluster{"x":dbl, "y":dbl, "w":dbl, "h":dbl} {"x"=4.0, "y"=4.0, "w"=-4.0, "h"=-4.0}) -> (x+y=w376:cluster{"x":dbl, "y":dbl, "w":dbl, "h":dbl})
              n154 = call <vilib>:"Draw Oval.vi"("picture"=w374, "rect"=w376, "fill?(F)"=TRUE, "color(black)"=w372) -> ("new picture"=w382:picture)  [unwired: 1 in, 4 out]
            }
            frame "<<Initial>>" {
              n155 = Select(t=u32 16318226, s=w386, f=u32 0) -> (s? t:f=w383:u32)
              n156 = call <vilib>:"Draw Oval.vi"("picture"=w388, "rect"=w390, "fill?(F)"=TRUE, "color(black)"=w383) -> ("new picture"=w389:picture)  [unwired: 1 in, 4 out]
            }
            frame Default {
              n157 = call <vilib>:"Draw Text in Rect.vi"("BG color(transparent)"=w397, "text color(black)"=u32 0, "text"=w394, "rect"=w391, "picture"=w396) -> ("new picture"=w393:picture)  [unwired: 3 in, 3 out]
              n158 = call <vilib>:"Draw Rect.vi"("picture"=w393, "rect"=w391) -> ("new picture"=w392:picture)  [unwired: 3 in, 4 out]
            }
          }
        }
        n159 = for {
          shift-right: [w339] -> w320
          shift-left: w325 -> [w340]
          tunnel: w324 -> [w350] mode=indexing
          tunnel: w323 -> [w349]
          n160 = Unbundle By Name(w350) -> ("len"=w327:dbl, "from"=w346:i32, "to"=w345:i32)
          n161 = Index Array(array=w349, index=w346) -> (element=w348:T21)
          n162 = Index Array(array=w349, index=w345) -> (element=w347:T21)
          n163 = Unbundle By Name(w348) -> ("x"=w338:dbl, "y"=w336:dbl)
          n164 = Unbundle By Name(w347) -> ("x"=w337:dbl, "y"=w335:dbl)
          n165 = Subtract(x=w338, y=w337) -> (x-y=w334:dbl)
          n166 = Subtract(x=w336, y=w335) -> (x-y=w333:dbl)
          n167 = Multiply(x=w334, y=w334) -> (x*y=w331:dbl)
          n168 = Multiply(x=w333, y=w333) -> (x*y=w332:dbl)
          n169 = Add(x=w331, y=w332) -> (x+y=w330:dbl)
          n170 = Square Root(x=w330) -> (sqrt(x)=w328:dbl)
          n171 = Subtract(x=w328, y=w327) -> (x-y=w329:dbl)
          n172 = Bundle("x"=w338, "y"=w336) -> (w344:cluster{"x":dbl, "y":dbl})  [unwired: 1 out]
          n173 = Bundle("x"=w337, "y"=w335) -> (w343:cluster{"x":dbl, "y":dbl})  [unwired: 1 out]
          n174 = case shown="20..29" w329 {
            tunnel: [u32 0 u32 16769042 u32 16745472 u32 16714752 u32 11250603] -> w341
            frame -9..9 {
            }
            frame 10..19 {
            }
            frame 20..29 {
            }
            frame 30.. {
            }
            frame Default {
            }
          }
          n175 = Build Array(w344, w343) -> (w342:cluster{"x":dbl, "y":dbl}[])
          n176 = call <vilib>:"Draw Multiple Lines.vi"("picture"=w340, "line endpoints"=w342, "color(black)"=w341) -> ("new picture"=w339:picture)  [unwired: 2 in, 4 out]
        }
        "Picture" <- w320
      }
      frame "GetUserInput" {
        n177 = event shown="[12] \"cancel\", \"OK\": Value Change" {
          selector: w398 -> [_ _ _ _ _ _ _ _ _ _ _ _ _]
          dyn-events: _ -> [_ _ _ _ _ _ _ _ _ _ _ _ _]
          timeout: 100 -> [_ _ _ _ _ _ _ _ _ _ _ _ _]
          tunnel: [w422 w461 w467 w474 w496 w510 w512 w514 w518 w543 w570 w573 w578] -> w405
          tunnel: w404 -> [w421 w461 w467 w474 w501 w510 w512 w514 w517 w544 w570 w573 w579]
          tunnel: [_ _ _ w475 "Paint" "Increase" "Decrease" "Shake" _ _ _ _ w580] -> w399
          event "Picture": Mouse Down {
            w406 = 1 ("y")
            n178 = event-data() -> ("Button"=w419:u16)  [unwired: 1 out]
            n179 = Unbundle By Name(w421) -> ("nodes"=w418:T20)
            n180 = property on="Picture" class="Pict"() -> ("Mouse"=w412:T24)  [unwired: 2 in, 2 out]
            n181 = property on="Picture" class="Pict" props=["Zoom Factor"]() -> ()  [unwired: 2 in, 3 out]
            n182 = Unbundle By Name(w412) -> ("Mouse Position.X"=w409:i32, "Mouse Position.Y"=w410:i32)
            n183 = Divide(x=w410, y=w406) -> (x/y=w407:dbl)
            n184 = Divide(x=w409, y=w406) -> (x/y=w408:dbl)
            n185 = Bundle(w408, w407) -> (w411:cluster{dbl, dbl})  [unwired: 1 out]
            n186 = for {
              tunnel: w418 -> [w427] mode=indexing
              tunnel: w411 -> [w425]
              tunnel: [w424] -> w417 mode=indexing
              tunnel: [w423] -> w415
              i -> [w423]
              n187 = call <resource>:"ArrangeNodes ConvertNodeDataToBounds.vi"("NodeData"=w427) -> ("NodeBounds"=w426:cluster{"x":dbl, "y":dbl, "w":dbl, "h":dbl})
              n188 = call <resource>:"Rectangel ContainsInBound.vi"("point2D"=w425, "bounds"=w426) -> ("contains"=w424:bool)  [unwired: 2 in, 15 out]
            }
            n189 = Reverse 1D Array(array=w417) -> (reversed array=w416:bool[])
            n190 = Search 1D Array(1D array=w416, element=TRUE) -> (index of element=w414:i32)  [unwired: 1 out]
            n191 = Subtract(x=w415, y=w414) -> (x-y=w413:i32)
            n192 = case shown="Default" w413 {
              selector: w413 -> [w429 _]
              tunnel: w421 -> [w432 w458]
              tunnel: [w428 w457] -> w422
              tunnel: w419 -> [w430 _]
              tunnel: w411 -> [w431 _]
              frame Default {
                n193 = case shown="0, Default" w430 {
                  tunnel: w432 -> [w441 w452]
                  tunnel: w431 -> [_ w448]
                  tunnel: w429 -> [w434 w447]
                  tunnel: [w433 w446] -> w428
                  frame 2 {
                    n194 = Unbundle By Name(w441) -> ("nodes"=w438:T20)
                    n195 = Index Array(array=w438, index=w434) -> (element=w437:T21)
                    n196 = Unbundle By Name(w437) -> ("fixed"=w436:bool)
                    n197 = Not(x=w436) -> (.not. x?=w435:bool)
                    n198 = Bundle By Name(cluster=w437, "fixed"=w435) -> (w443:T21)
                    n199 = Replace Array Subset(array=w438, new element=w443, index=w434) -> (w442:T20)
                    n200 = Bundle By Name(cluster=w441, "drag"=FALSE, "nodeSelected"=-1, "nodes"=w442) -> (w433:T14)
                  }
                  frame 0, Default {
                    n201 = Unbundle By Name(w452) -> ("nodes"=w450:T20)
                    n202 = Index Array(array=w450, index=w447) -> (element=w445:T21)
                    n203 = Bundle By Name(cluster=w445, "fixed"=TRUE) -> (w454:T21)
                    n204 = Unbundle By Name(w445) -> ("fixed"=w444:bool)
                    n205 = Replace Array Subset(array=w450, new element=w454, index=w447) -> (w453:T20)
                    n206 = Bundle By Name(cluster=w452, "fixedBeforeDrag"=w444, "drag"=TRUE, "nodeSelected"=w447, "DragStart"=w448, "nodes"=w453) -> (w446:T14)
                  }
                }
              }
              frame -1 {
                n207 = Bundle By Name(cluster=w458, "nodeSelected"=-1, "drag"=FALSE) -> (w457:T14)
              }
            }
          }
          event "Zoom": Value Change {
            n208 = event-data() -> ()  [unwired: 7 out]
            n209 = case shown="\"Smaller\"" "Zoom" {
              tunnel: [sgl 1.0 ("Zoom Factor") sgl 0.75 ("Zoom Factor") sgl 0.5 ("Zoom Factor") sgl 0.25 ("Zoom Factor")] -> w459
              frame "Normal", Default {
              }
              frame "Small" {
              }
              frame "Smaller" {
              }
              frame "Smallest" {
              }
            }
            n210 = property on="Picture" class="Pict"("Zoom Factor"=w459) -> ()  [unwired: 2 in, 2 out]
          }
          event "Auto Zoom": Value Change {
            n211 = event-data() -> ()  [unwired: 7 out]
            n212 = case shown="False" "Auto Zoom" {
              frame False {
                n213 = local read "Zoom"() -> (w469:enum16{"Normal", "Small", "Smaller", "Smallest"})
                n214 = case shown="\"Smallest\"" w469 {
                  tunnel: [sgl 1.0 ("Zoom Factor") sgl 0.75 ("Zoom Factor") sgl 0.5 ("Zoom Factor") sgl 0.25 ("Zoom Factor")] -> w468
                  frame "Normal", Default {
                  }
                  frame "Small" {
                  }
                  frame "Smaller" {
                  }
                  frame "Smallest" {
                  }
                }
                n215 = property on="Picture" class="Pict"("Zoom Factor"=w468) -> ()  [unwired: 2 in, 2 out]
              }
              frame True {
              }
            }
          }
          event "shorten": Value Change {
            n216 = event-data() -> ()  [unwired: 2 out]
            n217 = Unbundle By Name(w474) -> ("nodes"=w478:T20)
            n218 = Array Size(array=w478) -> (size(s)=w480:i32)
            n219 = Decrement(x=w480) -> (x-1=w479:i32)
            n220 = for {
              N: w479 -> [_]
              tunnel: w478 -> [w486] mode=indexing
              tunnel: w478 -> [w488]
              tunnel: [w483] -> w477 mode=indexing
              i -> [w489]
              n221 = Increment(x=w489) -> (x+1=w490:i32)
              n222 = call <resource>:"ArrangeNodes ConvertNodeDataToBounds.vi"("NodeData"=w486) -> ("NodeBounds"=w485:cluster{"x":dbl, "y":dbl, "w":dbl, "h":dbl})
              n223 = Array Subset(array=w488, index=w490) -> (w487:T20)  [unwired: 1 in]
              n224 = for {
                tunnel: w487 -> [w494] mode=indexing
                tunnel: w485 -> [w492]
                tunnel: [w491] -> w484 mode=indexing
                n225 = call <resource>:"ArrangeNodes ConvertNodeDataToBounds.vi"("NodeData"=w494) -> ("NodeBounds"=w493:cluster{"x":dbl, "y":dbl, "w":dbl, "h":dbl})
                n226 = call <resource>:"Rectangel RectangleOverlap.vi"("bounds1"=w492, "bounds2"=w493) -> ("overlap"=w491:bool)  [unwired: 2 in, 15 out]
              }
              n227 = Or Array Elements(Boolean array=w484) -> (logical OR=w483:bool)
            }
            n228 = Or Array Elements(Boolean array=w477) -> (logical OR=w476:bool)
            n229 = case shown="False" w476 {
              tunnel: ["Shorten" _] -> w475
              frame False {
              }
              frame True {
                n230 = One Button Dialog(message="Only allowed if non of the\nnodes are overlaping.") -> ()  [unwired: 2 out]
              }
            }
          }
          event "Min Length", "Max Length": Value Change {
            n231 = event-data() -> ()  [unwired: 4 out]
            n232 = Greater?(x="Min Length", y="Max Length") -> (0:w500:bool)
            n233 = Select(t="Min Length", s=w500, f="Max Length") -> (s? t:f=w497:i32)
            n234 = local write "Max Length"(w497) -> ()
            n235 = Unbundle By Name(w501) -> ("edges"=w503:cluster{"from":i32, "to":i32, "len":dbl}[])
            n236 = for {
              tunnel: w503 -> [w509] mode=indexing
              tunnel: [w508] -> w502 mode=indexing
              tunnel: w497 -> [w505]
              tunnel: "Min Length" -> [w504]
              n237 = Unbundle By Name(w509) -> ("len"=w507:dbl)
              n238 = In Range and Coerce(upper limit=w505, x=w507, lower limit=w504) -> (coerced(x)=w506:dbl)  [unwired: 1 out]
              n239 = Bundle(cluster=w509, "len"=w506) -> (w508:cluster{"from":i32, "to":i32, "len":dbl})  [unwired: 2 in]
            }
            n240 = Bundle By Name(cluster=w501, "edges"=w502) -> (w496:T14)
          }
          event "increase": Value Change {
            n241 = event-data() -> ()  [unwired: 2 out]
          }
          event "decrease": Value Change {
            n242 = event-data() -> ()  [unwired: 2 out]
          }
          event "Shake": Value Change {
            n243 = event-data() -> ()  [unwired: 2 out]
          }
          event "Picture": Mouse Up {
            n244 = event-data() -> ()  [unwired: 3 out]
            n245 = Unbundle By Name(w517) -> ("nodeSelected"=w516:i32)
            n246 = case shown="0, Default" w516 {
              selector: w516 -> [w521 _]
              tunnel: [w526 w529] -> w518
              tunnel: w517 -> [w520 w529]
              frame 0, Default {
                n247 = Unbundle By Name(w520) -> ("fixedBeforeDrag"=w519:bool)
                n248 = Unbundle By Name(w520) -> ("nodes"=w524:T20)
                n249 = Index Array(array=w524, index=w521) -> (element=w523:T21)
                n250 = Bundle By Name(cluster=w523, "fixed"=w519) -> (w525:T21)
                n251 = Replace Array Subset(array=w524, new element=w525, index=w521) -> (w522:T20)
                n252 = Bundle By Name(cluster=w520, "nodeSelected"=-1, "drag"=FALSE, "nodes"=w522) -> (w526:T14)
              }
              frame -1 {
              }
            }
          }
          event Timeout {
            w533 = 1 ("y")
            n253 = event-data() -> ()  [unwired: 2 out]
            n254 = property on="Picture" class="Pict"() -> ("Mouse"=w542:T24)  [unwired: 2 in, 2 out]
            n255 = Unbundle By Name(w544) -> ("drag"=w546:bool, "nodeSelected"=w540:i32, "DragStart"=w538:cluster{"X":i32, "Y":i32})
            n256 = property on="Picture" class="Pict"() -> ("Origin:Left"=w536:i16, "Origin:Top"=w535:i16)  [unwired: 2 in, 2 out]
            n257 = property on="Picture" class="Pict" props=["Zoom Factor"]() -> ()  [unwired: 2 in, 3 out]
            n258 = Unbundle By Name(w542) -> ("Mouse Position.X"=w532:i32, "Mouse Position.Y"=w534:i32)
            n259 = Divide(x=w534, y=w533) -> (x/y=w530:dbl)
            n260 = Divide(x=w532, y=w533) -> (x/y=w531:dbl)
            n261 = property class="VI"("Front Panel Window:Is Frontmost"=TRUE) -> ()  [unwired: 2 in, 2 out]
            n262 = Bundle(w531, w530) -> (w539:cluster{dbl, dbl})  [unwired: 1 out]
            n263 = Greater Or Equal To 0?(x=w540) -> (x >= 0?=w547:bool)
            n264 = And(x=w546, y=w547) -> (x .and. y?=w545:bool)
            n265 = Subtract(x=w539, y=w538) -> (x-y=w541:cluster{dbl, dbl})
            n266 = case shown="True" w545 {
              tunnel: w544 -> [w549 w563]
              tunnel: [w548 w562] -> w543
              tunnel: w541 -> [_ w559]
              tunnel: w540 -> [_ w561]
              tunnel: w539 -> [_ w554]
              tunnel: w536 -> [_ _]
              tunnel: w535 -> [_ _]
              tunnel: w533 -> [_ _]
              frame False {
                n267 = Bundle By Name(cluster=w549, "nodeSelected"=-1, "drag"=FALSE) -> (w548:T14)
              }
              frame True {
                n268 = Unbundle(w559) -> (w553:dbl, w552:dbl)
                n269 = Unbundle By Name(w563) -> ("nodes"=w564:T20)
                n270 = Index Array(array=w564, index=w561) -> (element=w560:T21)
                n271 = Unbundle By Name(w560) -> ("x"=w558:dbl, "y"=w557:dbl)
                n272 = Add(x=w558, y=w553) -> (x+y=w556:dbl)
                n273 = Add(x=w557, y=w552) -> (x+y=w555:dbl)
                n274 = Bundle By Name(cluster=w560, "x"=w556, "y"=w555) -> (w565:T21)
                n275 = Replace Array Subset(array=w564, new element=w565, index=w561) -> (w566:T20)
                n276 = Bundle By Name(cluster=w563, "DragStart"=w554, "nodes"=w566) -> (w562:T14)
              }
            }
          }
          event "Help": Value Change {
            n277 = event-data() -> ()  [unwired: 2 out]
            n278 = case shown="True" "Help" {
              tunnel: [ContextHelp_HelpTexts."None(Hide)" ("HelpText") ContextHelp_HelpTexts."ArrangeNodes Main" ("HelpText")] -> w568
              frame False {
              }
              frame True {
              }
            }
            n279 = call <resource>:"ContextHelp_HelpTexts.vi"("HelpText (enum or string)"=w568) -> ("HelpOut"=w569:T25)  [unwired: 18 out]
            n280 = call <resource>:"ContextHelp_SendMessageToPopUp.vi"("PopUpMessage"=w569) -> ()  [unwired: 2 in, 17 out]
          }
          event Mouse Enter {
            n281 = event-data() -> ("CtlRef"=w575:refnum<vi>)  [unwired: 1 out]
            n282 = local read "Help"() -> (w574:bool)
            n283 = call <resource>:"ContextHelp_CheckHelpForControl.vi"("Ctl Refnum"=w575, "Help"=w574) -> ()  [unwired: 1 in, 17 out]
          }
          event "cancel", "OK": Value Change {
            n284 = event-data() -> ()  [unwired: 2 out]
            n285 = Bundle By Name(cluster=w579, "Cancel"="cancel") -> (w578:T14)
            n286 = case shown="True" "OK" {
              tunnel: ["Exit" "UpdateNodes"] -> w580
              frame False {
              }
              frame True {
              }
            }
          }
        }
        n287 = Empty String/Path?(string/path=w399) -> (empty?=w401:bool)
        n288 = Select(t="Simulate", s=w401, f=w399) -> (s? t:f=w403:string)
      }
      frame "Shorten" {
        n289 = local read "Min Length"() -> (w585:i32)
        n290 = call <vilib>:"Set Busy.vi"() -> ("error out"=w583:errorcluster)  [unwired: 4 in, 7 out]
        n291 = while {
          shift-right: [w599] -> w586
          shift-left: w587 -> [w591]
          tunnel: w585 -> [w590]
          tunnel: [w589] -> w584
          tunnel: w583 -> [w589]
          i -> [w596]
          stop <- w592 stop-if-true
          n292 = Unbundle By Name(w591) -> ("nodes"=w598:T20)
          n293 = Array Size(array=w598) -> (size(s)=w602:i32)
          n294 = Decrement(x=w602) -> (x-1=w601:i32)
          n295 = for {
            N: w601 -> [_]
            tunnel: w598 -> [w622] mode=indexing
            tunnel: w598 -> [w624]
            tunnel: [w619] -> w600 mode=indexing
            i -> [w625]
            n296 = Increment(x=w625) -> (x+1=w626:i32)
            n297 = call <resource>:"ArrangeNodes ConvertNodeDataToBounds.vi"("NodeData"=w622) -> ("NodeBounds"=w621:cluster{"x":dbl, "y":dbl, "w":dbl, "h":dbl})
            n298 = Array Subset(array=w624, index=w626) -> (w623:T20)  [unwired: 1 in]
            n299 = for {
              tunnel: w623 -> [w630] mode=indexing
              tunnel: w621 -> [w628]
              tunnel: [w627] -> w620 mode=indexing
              n300 = call <resource>:"ArrangeNodes ConvertNodeDataToBounds.vi"("NodeData"=w630) -> ("NodeBounds"=w629:cluster{"x":dbl, "y":dbl, "w":dbl, "h":dbl})
              n301 = call <resource>:"Rectangel RectangleOverlap.vi"("bounds1"=w628, "bounds2"=w629) -> ("overlap"=w627:bool)  [unwired: 2 in, 15 out]
            }
            n302 = Or Array Elements(Boolean array=w620) -> (logical OR=w619:bool)
          }
          n303 = Or Array Elements(Boolean array=w600) -> (logical OR=w593:bool)
          n304 = case shown="False" w593 {
            tunnel: w591 -> [w609 w618]
            tunnel: [w604 w618] -> w597
            tunnel: w590 -> [w603 _]
            frame False {
              n305 = Unbundle By Name(w609) -> ("edges"=w608:cluster{"from":i32, "to":i32, "len":dbl}[])
              n306 = for {
                tunnel: w608 -> [w617] mode=indexing
                tunnel: [w615] -> w607 mode=indexing
                tunnel: w603 -> [w612]
                n307 = Unbundle By Name(w617) -> ("len"=w616:dbl)
                n308 = Decrement(x=w616) -> (x-1=w613:dbl)
                n309 = Max & Min(x=w613, y=w612) -> (max(x,y)=w614:dbl)  [unwired: 1 out]
                n310 = Bundle(cluster=w617, "len"=w614) -> (w615:cluster{"from":i32, "to":i32, "len":dbl})  [unwired: 2 out]
              }
              n311 = Bundle By Name(cluster=w609, "edges"=w607) -> (w606:T14)
              n312 = for {
                N: 10 -> [_]
                shift-right: [w610] -> w604
                shift-left: w606 -> [w611]
                n313 = call <resource>:"ArrangeNodes SimulationSubVI.vi"("varIn"=w611) -> ("varOut"=w610:T14)  [unwired: 1 in, 17 out]
              }
            }
            frame True {
            }
          }
          n314 = Greater Or Equal?(x=w596, y=500) -> (x >= y?=w594:bool)
          n315 = Or(x=w594, y=w593) -> (x .or. y?=w592:bool)
          n316 = Select(t=w591, s=w593, f=w597) -> (s? t:f=w599:T14)
        }
        n317 = call <vilib>:"Unset Busy.vi"("error in (no error)"=w584) -> ()  [unwired: 1 in, 10 out]
      }
      frame "Shake" {
        n318 = while {
          shift-right: [w648] -> w634
          shift-left: w636 -> [w651]
          i -> [w645]
          stop <- w652 stop-if-true
          n319 = Unbundle By Name(w651) -> ("nodes"=w647:T20)
          n320 = Array Size(array=w647) -> (size(s)=w655:i32)
          n321 = Decrement(x=w655) -> (x-1=w654:i32)
          n322 = Equal To 0?(x=w645) -> (x = 0?=w646:bool)
          n323 = Select(t=1, s=w646, f=5) -> (s? t:f=w644:i32)
          n324 = for {
            N: w654 -> [_]
            tunnel: w647 -> [w665] mode=indexing
            shift-right: [w663] -> w649
            shift-left: w651 -> [w664]
            shift-right: [w660] -> _
            shift-left: w647 -> [w661]
            tunnel: w644 -> [w659]
            i -> [w662]
            n325 = Unbundle By Name(w665) -> ("fixed"=w666:bool)
            n326 = case shown="False" w666 {
              tunnel: w665 -> [w670 _]
              tunnel: w661 -> [w673 w720]
              tunnel: w664 -> [w672 w721]
              tunnel: [w671 w721] -> w663
              tunnel: w662 -> [w669 _]
              tunnel: [w668 w720] -> w660
              tunnel: w659 -> [w667 _]
              frame False {
                n327 = for {
                  N: w667 -> [_]
                  shift-right: [w686] -> w668
                  shift-left: w673 -> [w690]
                  shift-right: [w677] -> w671
                  shift-left: w672 -> [w685]
                  tunnel: w670 -> [w676]
                  tunnel: w669 -> [w679]
                  i -> [w684]
                  n328 = Unbundle By Name(w676) -> ("x"=w683:dbl, "y"=w678:dbl)
                  n329 = Unbundle By Name(w676) -> ("dx"=w675:dbl, "dy"=w674:dbl)
                  n330 = case shown="1" w684 {
                    tunnel: w683 -> [w702 w706 w710 w711 w714]
                    tunnel: [w701 w704 w708 w711 w714] -> w682
                    tunnel: [w699 w703 w707 w712 w715] -> w681
                    tunnel: w678 -> [w700 w703 w707 _ _]
                    tunnel: w675 -> [w698 _ _ _ _]
                    tunnel: w674 -> [w694 _ _ _ _]
                    frame 0, Default {
                      w692 = -50.0 ("f")
                      w693 = 50.0 ("t")
                      n331 = Greater Than 0?(x=w698) -> (x > 0?=w697:bool)
                      n332 = Greater Than 0?(x=w694) -> (x > 0?=w695:bool)
                      n333 = Select(t=w693, s=w697, f=w692) -> (s? t:f=w696:dbl)
                      n334 = Select(t=w693, s=w695, f=w692) -> (s? t:f=w691:dbl)
                      n335 = Add(x=w702, y=w696) -> (x+y=w701:dbl)
                      n336 = Add(x=w700, y=w691) -> (x+y=w699:dbl)
                    }
                    frame 1 {
                      n337 = Add(x=w706, y=5.0) -> (x+y=w704:dbl)
                    }
                    frame 2 {
                      n338 = Subtract(x=w710, y=10.0) -> (x-y=w708:dbl)
                    }
                    frame 3 {
                      n339 = Subtract(x=w711, y=5.0) -> (x-y=w712:dbl)
                    }
                    frame 4 {
                      n340 = Add(x=w714, y=10.0) -> (x+y=w715:dbl)
                    }
                  }
                  n341 = Bundle By Name(cluster=w676, "x"=w682, "y"=w681) -> (w680:T21)
                  n342 = Replace Array Subset(array=w690, new element=w680, index=w679) -> (w688:T20)
                  n343 = Bundle By Name(cluster=w685, "nodes"=w688) -> (w687:T14)
                  n344 = for {
                    N: 5 -> [_]
                    shift-right: [w718] -> w677
                    shift-left: w687 -> [w719]
                    n345 = call <resource>:"ArrangeNodes SimulationSubVI.vi"("varIn"=w719, "AllowOverlap(False)"=TRUE) -> ("varOut"=w718:T14)  [unwired: 17 out]
                  }
                  n346 = Unbundle By Name(w677) -> ("nodes"=w686:T20)
                }
              }
              frame True {
              }
            }
          }
          n347 = Greater?(x=w645, y=1) -> (0:w652:bool)
          n348 = for {
            N: 5 -> [_]
            shift-right: [w657] -> w648
            shift-left: w649 -> [w658]
            n349 = call <resource>:"ArrangeNodes SimulationSubVI.vi"("varIn"=w658, "AllowOverlap(False)"=TRUE) -> ("varOut"=w657:T14)  [unwired: 17 out]
          }
        }
        n350 = call <vilib>:"Set Busy.vi"() -> ("error out"=w631:errorcluster)  [unwired: 4 in, 7 out]
        n351 = for {
          N: 5 -> [_]
          shift-right: [w640] -> w633
          shift-left: w634 -> [w641]
          tunnel: [w638] -> w632
          tunnel: w631 -> [w638]
          n352 = call <resource>:"ArrangeNodes SimulationSubVI.vi"("varIn"=w641, "AllowOverlap(False)"=FALSE) -> ("varOut"=w640:T14)  [unwired: 17 out]
        }
        n353 = call <vilib>:"Unset Busy.vi"("error in (no error)"=w632) -> ()  [unwired: 1 in, 10 out]
      }
      frame "Old Shake" {
        n354 = while {
          shift-right: [w728] -> w722
          shift-left: w723 -> [w729]
          i -> [w727]
          stop <- w725 stop-if-true
          n355 = Unbundle By Name(w729) -> ("nodes"=w730:T20)
          n356 = Array Size(array=w730) -> (size(s)=w732:i32)
          n357 = Decrement(x=w732) -> (x-1=w731:i32)
          n358 = for {
            N: w731 -> [_]
            tunnel: w730 -> [w737] mode=indexing
            tunnel: w730 -> [w736]
            shift-right: [w734] -> w728
            shift-left: w729 -> [w735]
            i -> [w733]
            n359 = Unbundle By Name(w737) -> ("fixed"=w738:bool)
            n360 = case shown="False" w738 {
              tunnel: w737 -> [w740 _]
              tunnel: w736 -> [w743 _]
              tunnel: w735 -> [w742 w776]
              tunnel: [w741 w776] -> w734
              tunnel: w733 -> [w739 _]
              frame False {
                n361 = for {
                  N: 4 -> [_]
                  shift-right: [w755] -> _
                  shift-left: w743 -> [w759]
                  shift-right: [w745] -> w741
                  shift-left: w742 -> [w754]
                  tunnel: w740 -> [w751]
                  tunnel: w739 -> [w747]
                  i -> [w753]
                  n362 = Unbundle By Name(w751) -> ("x"=w752:dbl, "y"=w746:dbl)
                  n363 = case shown="2" w753 {
                    tunnel: w752 -> [w763 w767 w768 w771]
                    tunnel: [w761 w765 w768 w771] -> w750
                    tunnel: [w760 w764 w769 w772] -> w749
                    tunnel: w746 -> [w760 w764 _ _]
                    frame 0, Default {
                      n364 = Add(x=w763, y=5.0) -> (x+y=w761:dbl)
                    }
                    frame 1 {
                      n365 = Subtract(x=w767, y=10.0) -> (x-y=w765:dbl)
                    }
                    frame 2 {
                      n366 = Subtract(x=w768, y=5.0) -> (x-y=w769:dbl)
                    }
                    frame 3 {
                      n367 = Add(x=w771, y=10.0) -> (x+y=w772:dbl)
                    }
                  }
                  n368 = Bundle By Name(cluster=w751, "x"=w750, "y"=w749) -> (w748:T21)
                  n369 = Replace Array Subset(array=w759, new element=w748, index=w747) -> (w757:T20)
                  n370 = Bundle By Name(cluster=w754, "nodes"=w757) -> (w756:T14)
                  n371 = for {
                    N: 5 -> [_]
                    shift-right: [w774] -> w745
                    shift-left: w756 -> [w775]
                    n372 = call <resource>:"ArrangeNodes SimulationSubVI.vi"("varIn"=w775) -> ("varOut"=w774:T14)  [unwired: 1 in, 17 out]
                  }
                  n373 = Unbundle By Name(w745) -> ("nodes"=w755:T20)
                }
              }
              frame True {
              }
            }
          }
          n374 = Greater?(x=w727, y=5) -> (0:w725:bool)
        }
      }
      frame "Increase" {
        n375 = local read "Max Length"() -> (w777:i32)
        n376 = Unbundle By Name(w779) -> ("edges"=w781:cluster{"from":i32, "to":i32, "len":dbl}[])
        n377 = for {
          tunnel: w781 -> [w789] mode=indexing
          tunnel: [w788] -> w780 mode=indexing
          tunnel: w777 -> [w784]
          n378 = Unbundle By Name(w789) -> ("len"=w787:dbl)
          n379 = Add(x=w787, y=5.0) -> (x+y=w785:dbl)
          n380 = Max & Min(x=w785, y=w784) -> (min(x,y)=w783:dbl)  [unwired: 1 out]
          n381 = Bundle(cluster=w789, "len"=w783) -> (w788:cluster{"from":i32, "to":i32, "len":dbl})  [unwired: 2 in]
        }
        n382 = Bundle By Name(cluster=w779, "edges"=w780) -> (w778:T14)
      }
      frame "Decrease" {
        n383 = local read "Min Length"() -> (w790:i32)
        n384 = Unbundle By Name(w792) -> ("edges"=w794:cluster{"from":i32, "to":i32, "len":dbl}[])
        n385 = for {
          tunnel: w794 -> [w802] mode=indexing
          tunnel: [w801] -> w793 mode=indexing
          tunnel: w790 -> [w797]
          n386 = Unbundle By Name(w802) -> ("len"=w800:dbl)
          n387 = Subtract(x=w800, y=5.0) -> (x-y=w798:dbl)
          n388 = Max & Min(x=w798, y=w797) -> (max(x,y)=w796:dbl)  [unwired: 1 out]
          n389 = Bundle(cluster=w802, "len"=w796) -> (w801:cluster{"from":i32, "to":i32, "len":dbl})  [unwired: 2 in]
        }
        n390 = Bundle By Name(cluster=w792, "edges"=w793) -> (w791:T14)
      }
      frame "Simulate" {
        n391 = call <resource>:"ArrangeNodes SimulationSubVI.vi"("varIn"=w805) -> ("varOut"=w804:T14)  [unwired: 1 in, 17 out]
      }
      frame "Offset" {
        w829 = dbl[] []
        w836 = 250.0 ("y")
        w842 = 2.0 ("y")
        n392 = Unbundle By Name(w832) -> ("nodes"=w847:T20)
        n393 = for {
          tunnel: w847 -> [w874] mode=indexing
          shift-right: [w883] -> w830
          shift-left: w829 -> [w885]
          shift-right: [w882] -> w828
          shift-left: w829 -> [w884]
          tunnel: [w881] -> w827 mode=indexing
          tunnel: [w880] -> w824 mode=indexing
          tunnel: [w877] -> w817 mode=indexing
          tunnel: [w872] -> w811 mode=indexing
          tunnel: [w871] -> w810 mode=indexing
          n394 = Unbundle By Name(w874) -> ("w"=w879:dbl, "h"=w878:dbl, "x"=w876:dbl, "y"=w875:dbl, "fixed"=w881:bool)
          n395 = Add(x=w879, y=w876) -> (x+y=w880:dbl)
          n396 = Add(x=w878, y=w875) -> (x+y=w877:dbl)
          n397 = case shown="False" w881 {
            tunnel: w876 -> [w891 _]
            tunnel: w875 -> [w888 _]
            tunnel: [w889 w893] -> w883
            tunnel: [w886 w892] -> w882
            tunnel: w885 -> [w890 w893]
            tunnel: w884 -> [w887 w892]
            frame False {
              n398 = Build Array (concatenate)(w890, w891) -> (w889:dbl[])
              n399 = Build Array (concatenate)(w887, w888) -> (w886:dbl[])
            }
            frame True {
            }
          }
          n400 = call <resource>:"ArrangeNodes ConvertNodeDataToBounds.vi"("NodeData"=w874) -> ("NodeBounds"=w873:cluster{"x":dbl, "y":dbl, "w":dbl, "h":dbl})
          n401 = Unbundle By Name(w873) -> ("x"=w872:dbl, "y"=w871:dbl)
        }
        n402 = property on="Picture" class="Pict"() -> ("Draw Area Size"=w823:T26)  [unwired: 2 in, 2 out]
        n403 = Unbundle By Name(w823) -> ("Width"=w822:u32, "Height"=w816:u32)
        n404 = Array Max & Min(array=w824) -> (max value=w818:dbl)  [unwired: 3 out]
        n405 = Array Max & Min(array=w817) -> (max value=w815:dbl)  [unwired: 3 out]
        n406 = Search 1D Array(1D array=w827, element=TRUE) -> (index of element=w825:i32)  [unwired: 1 out]
        n407 = Divide(x=w822, y=w818) -> (x/y=w821:dbl)
        n408 = Divide(x=w816, y=w815) -> (x/y=w813:dbl)
        n409 = Array Max & Min(array=w811) -> (min value=w807:dbl)  [unwired: 3 out]
        n410 = Array Max & Min(array=w810) -> (min value=w806:dbl)  [unwired: 3 out]
        n411 = Max & Min(x=w813, y=1.0) -> (min(x,y)=w812:dbl)  [unwired: 1 out]
        n412 = Array Max & Min(array=w830) -> (max value=w846:dbl, min value=w844:dbl)  [unwired: 2 out]
        n413 = Array Max & Min(array=w828) -> (max value=w845:dbl, min value=w839:dbl)  [unwired: 2 out]
        n414 = Subtract(x=w846, y=w844) -> (x-y=w843:dbl)
        n415 = Subtract(x=w845, y=w839) -> (x-y=w841:dbl)
        n416 = Divide(x=w843, y=w842) -> (x/y=w840:dbl)
        n417 = Divide(x=w841, y=w842) -> (x/y=w838:dbl)
        n418 = Max & Min(x=w821, y=w812) -> (min(x,y)=w820:dbl)  [unwired: 1 out]
        n419 = Add(x=w844, y=w840) -> (x+y=w837:dbl)
        n420 = Add(x=w839, y=w838) -> (x+y=w835:dbl)
        n421 = Subtract(x=w836, y=w837) -> (x-y=w834:dbl)
        n422 = Subtract(x=w836, y=w835) -> (x-y=w833:dbl)
        n423 = local read "Auto Zoom"() -> (w819:bool)
        n424 = case shown="-10" w825 {
          tunnel: w847 -> [w858 w862]
          tunnel: w834 -> [_ w861]
          tunnel: w833 -> [_ w860]
          tunnel: [w858 w859] -> w809
          frame Default {
          }
          frame -10 {
            n425 = for {
              tunnel: w862 -> [w866] mode=indexing
              tunnel: w861 -> [w869]
              tunnel: w860 -> [w867]
              tunnel: [w863] -> w859 mode=indexing
              n426 = Unbundle By Name(w866) -> ("x"=w870:dbl, "y"=w868:dbl)
              n427 = Add(x=w870, y=w869) -> (x+y=w865:dbl)
              n428 = Add(x=w868, y=w867) -> (x+y=w864:dbl)
              n429 = Bundle By Name(cluster=w866, "x"=w865, "y"=w864) -> (w863:T21)
            }
          }
        }
        n430 = case shown="False" w819 {
          tunnel: w820 -> [_ w857]
          frame False {
          }
          frame True {
            n431 = property on="Picture" class="Pict"("Zoom Factor"=w857) -> ()  [unwired: 2 in, 2 out]
          }
        }
        n432 = for {
          tunnel: w809 -> [w854] mode=indexing
          tunnel: [w851] -> w808 mode=indexing
          tunnel: w807 -> [w850]
          tunnel: w806 -> [w849]
          n433 = Unbundle By Name(w854) -> ("x"=w856:dbl, "y"=w855:dbl)
          n434 = Subtract(x=w856, y=w850) -> (x-y=w853:dbl)
          n435 = Subtract(x=w855, y=w849) -> (x-y=w852:dbl)
          n436 = Bundle By Name(cluster=w854, "x"=w853, "y"=w852) -> (w851:T21)
        }
        n437 = Bundle By Name(cluster=w832, "nodes"=w808) -> (w831:T14)
      }
      frame "UpdateNodes" {
        w896 = 10
        n438 = Unbundle By Name(w905) -> ("nodes"=w903:T20, "ClassNodes"=w904:refnum<class "AbstractNode.lvclass">[])
        n439 = for {
          tunnel: w903 -> [w914] mode=indexing
          tunnel: [w908] -> w902 mode=indexing
          tunnel: [w907] -> w897 mode=indexing
          n440 = Unbundle By Name(w914) -> ("x"=w913:dbl, "y"=w911:dbl, "w"=w912:dbl, "h"=w910:dbl)
          n441 = expression code="x/2"(w910) -> (w909:dbl)
          n442 = expression code="x/2"(w912) -> (w915:dbl)
          n443 = Subtract(x=w913, y=w915) -> (x-y=w908:dbl)
          n444 = Subtract(x=w911, y=w909) -> (x-y=w907:dbl)
        }
        n445 = Array Max & Min(array=w902) -> (min value=w901:dbl)  [unwired: 3 out]
        n446 = Array Max & Min(array=w897) -> (min value=w898:dbl)  [unwired: 3 out]
        n447 = Subtract(x=w902, y=w901) -> (x-y=w900:dbl[])
        n448 = Subtract(x=w897, y=w898) -> (x-y=w899:dbl[])
        n449 = Add(x=w900, y=w896) -> (x+y=w894:dbl[])
        n450 = Add(x=w899, y=w896) -> (x+y=w895:dbl[])
        n451 = for {
          tunnel: w904 -> [w916] mode=indexing
          tunnel: w894 -> [w918] mode=indexing
          tunnel: w895 -> [w917] mode=indexing
          n452 = call-dynamic "getBounds.vi"("reference"=w916) -> ("reference out"=w925:refnum<class "AbstractNode.lvclass">, "bounds"=w923:T7, "error out"=w924:errorcluster)  [unwired: 16 in]
          n453 = Unbundle By Name(w923) -> ("x"=w922:dbl, "y"=w920:dbl)
          n454 = Subtract(x=w918, y=w922) -> (x-y=w921:dbl)
          n455 = Subtract(x=w917, y=w920) -> (x-y=w919:dbl)
          n456 = call-dynamic "translate.vi"("reference"=w925, "dx"=w921, "dy"=w919, "error in (no error)"=w924) -> ()  [unwired: 14 in, 2 out]
        }
      }
    }
    n457 = Not Equal?(x=w18, y="Exit") -> (x != y?=w19:bool)
  }
  n458 = call <resource>:"CommonVIs_CloseControlRefs.vi"("Event Registration Refnum"=w4, "ControlRefs"=w8) -> ("error out"=w7:errorcluster)  [unwired: 1 in, 16 out]
  n459 = call <resource>:"ContextHelp_LeavingDialog.vi"("error in (no error)"=w7) -> ()  [unwired: 2 in, 17 out]
  n460 = Unbundle By Name(w2) -> ("Cancel"=→"Cancel":bool)
